vi "Set Theme Data From Caller.vi"(8 "Error In":errorcluster, 10 "Caller Appearance Actor in":refnum<class "Appearance Actor.lvclass">, 11 "Appearance Actor in":refnum<class "Appearance Actor.lvclass">) -> (0 "Error Out":errorcluster, 3 "Appearance Actor out":refnum<class "Appearance Actor.lvclass">)   [LabVIEW 2021, in "Appearance Actor.lvlib" / "Appearance Actor.lvclass"]
uses:
  Appearance Actor.lvclass
  Appearance Actor.lvclass/Appearance Actor.ctl
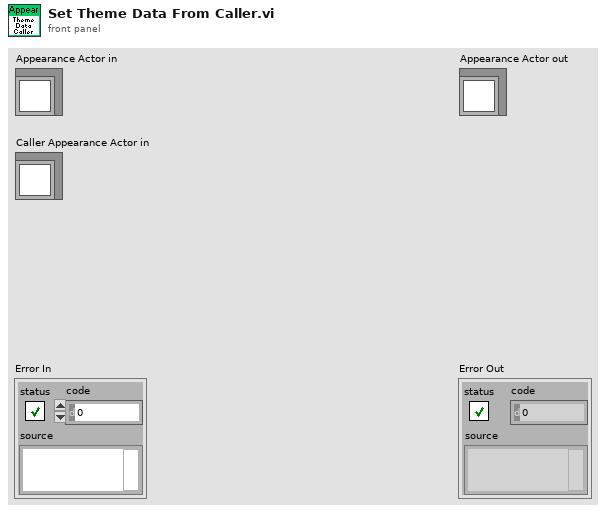
[diagram p1: front panel]
types:
  T1 = typedef "Appearance Actor.lvlib/Appearance Actor.lvclass/Theme Data--cluster.ctl" = cluster{"ini Config Ref":T2}
  T2 = typedef "NI_LVConfig.lvlib/Config Data RefNum.ctl" = refnum<k1>
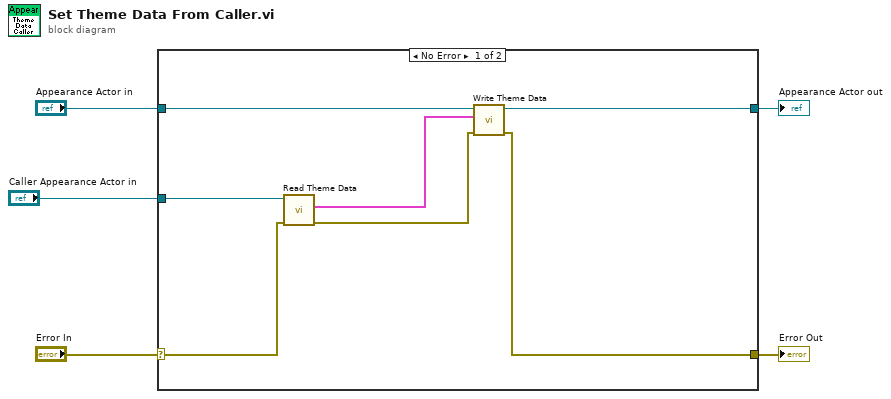
[diagram p0: block diagram]
diagram:
  n1 = case shown="No Error" "Error In" {
    selector: "Error In" -> [w8 w14]
    tunnel: [w6 w14] -> w4
    tunnel: [w11 w13] -> w2
    tunnel: "Appearance Actor in" -> [w12 w13]
    tunnel: "Caller Appearance Actor in" -> [w9 _]
    frame No Error {
      n2 = call "Read Theme Data.vi"("error in (no error)"=w8, "Appearance Actor in"=w9) -> ("error out"=w7:errorcluster, "Theme Data"=w10:T1)  [unwired: 7 in, 1 out]
      n3 = call "Write Theme Data.vi"("error in (no error)"=w7, "Theme Data"=w10, "Appearance Actor in"=w12) -> ("error out"=w6:errorcluster, "Appearance Actor out"=w11:refnum<class "Appearance Actor.lvclass">)  [unwired: 7 in]
    }
    frame Error {
    }
  }
  "Error Out" <- w4
  "Appearance Actor out" <- w2
